vi "Msg To.vi"(9 "Insert (T) or Remove (F)":bool, 10 "Queue Nested":map{string, refnum<data-value>}(c390)) -> (3 "Update Queue Nested Msg Strategy out":refnum<class "Update Queue Nested Msg Strategy.lvclass">)   [LabVIEW 2021, in "jettl.lvlib" / "Update Queue Nested.lvlib"]
uses:
  Update Queue Nested.lvlib
  Msg Strategy/Msg Strategy.lvclass
  Update Queue Nested Msg Strategy/Update Queue Nested Msg Strategy.lvclass
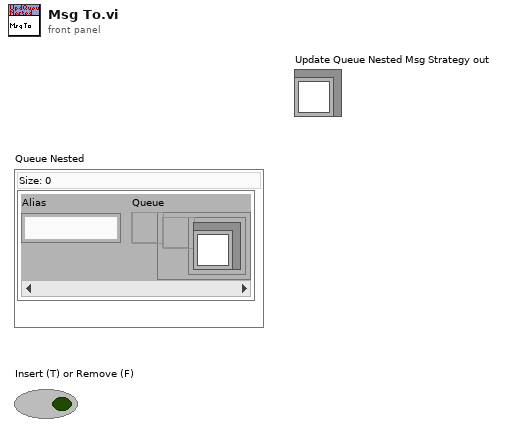
[diagram p1: front panel]
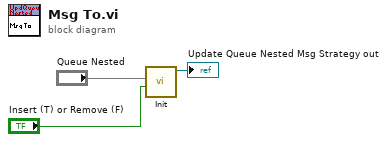
[diagram p0: block diagram]
diagram:
  n1 = call "Init.vi"("Insert (T) or Remove (F)"="Insert (T) or Remove (F)", "Queue Nested"="Queue Nested") -> ("Update Queue Nested Msg Strategy out"=→"Update Queue Nested Msg Strategy out":refnum<class "Update Queue Nested Msg Strategy.lvclass">)  [unwired: 9 in]
